vi "WebCam.Example03.vi"() -> ()   [LabVIEW 2021]
panel:
  out "snapshot 2":picture
  out "snapshot":picture
  in  "Case Constant\n(See Context Help)":bool
  in  "stop":bool
  out "error out":errorcluster
  in  "error in (no error)":errorcluster
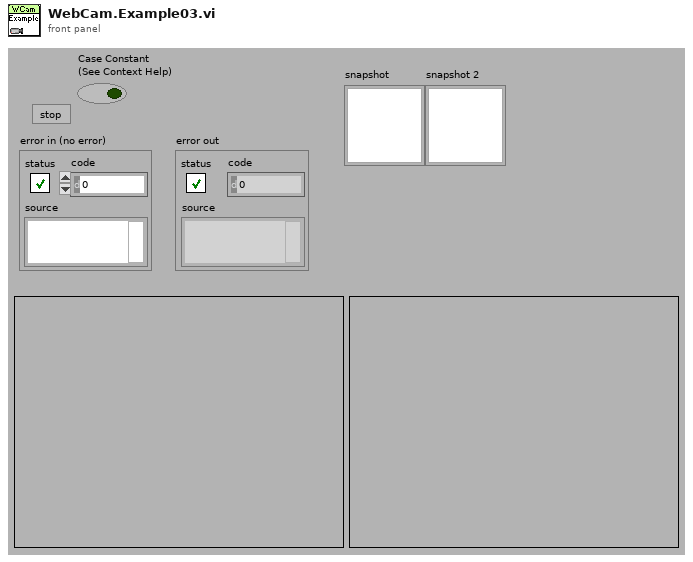
[diagram p1: front panel]
types:
  T1 = cluster{"posX":i32, "posY":i32, "nWidth":i32, "nHeight":i32}
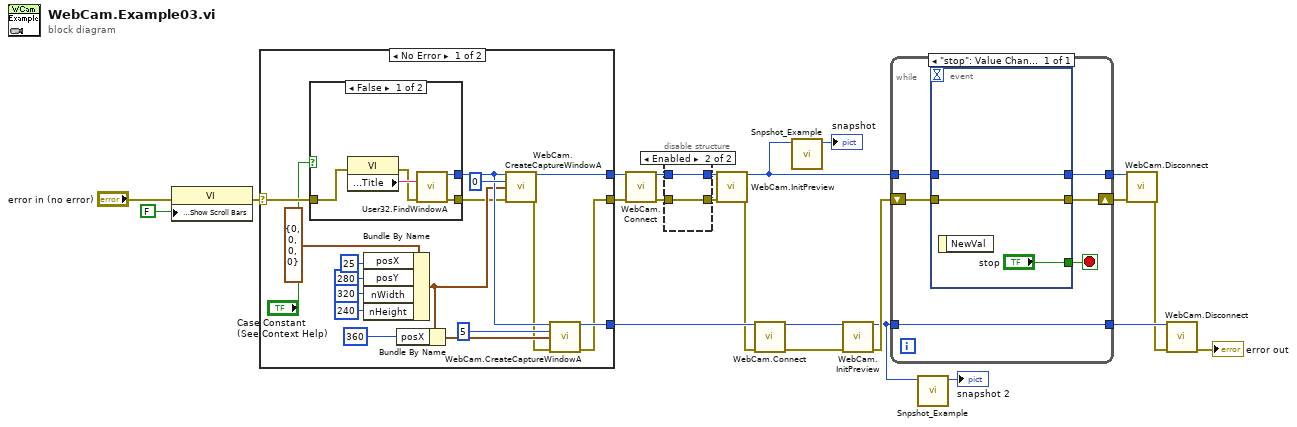
[diagram p0: block diagram]
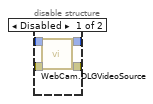
[diagram p2: hidden frame]
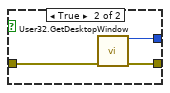
[diagram p3: hidden frame]
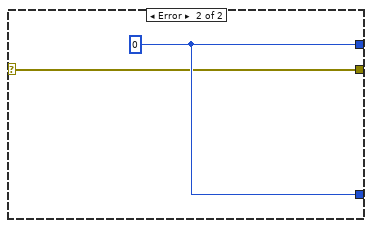
[diagram p4: hidden frame]
diagram:
  n1 = property class="VI"(error in="error in (no error)", "Front Panel Window:Show Scroll Bars"=FALSE) -> (error out=w20:errorcluster)  [unwired: 1 in, 1 out]
  n2 = case shown="No Error" w20 {
    selector: w20 -> [w40 w50]
    tunnel: [w41 w51] -> w15
    tunnel: [w24 w50] -> w14
    tunnel: [w30 w51] -> w18
    frame No Error {
      n3 = case shown="False" "Case Constant\n(See Context Help)" {
        tunnel: w40 -> [w43 w49]
        tunnel: [w46 w48] -> w33
        tunnel: [w45 w47] -> w25
        frame False {
          n4 = property class="VI"(error in=w43) -> (error out=w42:errorcluster, "Front Panel Window:Title"=w44:string)  [unwired: 1 in, 1 out]
          n5 = call "User32.FindWindowA.vi"("lpWindowName"=w44, "error in (no error)"=w42) -> ("hwnd"=w46:i32, "error out"=w45:errorcluster)  [unwired: 12 in]
        }
        frame True {
          n6 = call "User32.GetDesktopWindow.vi"("error in (no error)"=w49) -> ("Desktop handle"=w48:i32, "error out"=w47:errorcluster)  [unwired: 13 in]
        }
      }
      n7 = Bundle By Name(cluster=T1 {"posX"=0, "posY"=0, "nWidth"=0, "nHeight"=0} ("rect"), "posX"=25 ("nWidth"), "posY"=280 ("nWidth"), "nWidth"=320, "nHeight"=240 ("nWidth")) -> (w31:T1)
      n8 = Bundle By Name(cluster=w31, "posX"=360) -> (w28:T1)
      n9 = call "WebCam.CreateCaptureWindowA.vi"("handle"=w33, "nID"=0, "rect"=w31, "error in (no error)"=w25) -> ("handle out"=w41:i32, "error out"=w26:errorcluster)  [unwired: 10 in]
      n10 = call "WebCam.CreateCaptureWindowA.vi"("handle"=w33, "nID"=5, "rect"=w28, "error in (no error)"=w26) -> ("handle out"=w30:i32, "error out"=w24:errorcluster)  [unwired: 10 in]
    }
    frame Error {
      w51 = 0
    }
  }
  n11 = call "WebCam.Connect.vi"("handle"=w15, "error in (no error)"=w14) -> ("handle out"=w12:i32, "error out"=w11:errorcluster)  [unwired: 12 in]
  n12 = disable-structure shown="Enabled" {
    disable-tunnel: w12 -> [w55 w56]
    disable-tunnel: w11 -> [w54 w57]
    disable-tunnel: [w53 w57] -> w10
    disable-tunnel: [w52 w56] -> w9
    frame Disabled {
      n13 = call "WebCam.DLGVideoSource.vi"("handle"=w55, "error in (no error)"=w54) -> ("handle out"=w52:i32, "error out"=w53:errorcluster)  [unwired: 12 in]
    }
    frame Enabled {
    }
  }
  n14 = call "WebCam.InitPreview.vi"("handle"=w9, "error in (no error)"=w10) -> ("handle out"=w4:i32, "error out"=w8:errorcluster)  [unwired: 12 in]
  n15 = call "WebCam.Connect.vi"("handle"=w18, "error in (no error)"=w8) -> ("handle out"=w6:i32, "error out"=w5:errorcluster)  [unwired: 12 in]
  n16 = call "Snpshot_Example.vi"("handle"=w4) -> ("handle out"=→"snapshot":i32)  [unwired: 8 in, 2 out]
  n17 = call "WebCam.InitPreview.vi"("handle"=w6, "error in (no error)"=w5) -> ("handle out"=w1:i32, "error out"=w7:errorcluster)  [unwired: 12 in]
  n18 = while {
    shift-right: [w63] -> w23
    shift-left: w7 -> [w62]
    tunnel: w4 -> [w60]
    tunnel: [w59] -> w22
    tunnel: w1 -> [w58]
    tunnel: [w58] -> w17
    stop <- w61 stop-if-true
    n19 = event shown="[0] \"stop\": Value Change" {
      selector: _ -> [_]
      dyn-events: _ -> [_]
      timeout: _ -> [_]
      tunnel: [w66] -> w63
      tunnel: w62 -> [w66]
      tunnel: ["stop"] -> w61
      tunnel: w60 -> [w64]
      tunnel: [w64] -> w59
      event "stop": Value Change {
        n20 = event-data() -> ()  [unwired: 1 in, 1 out]
      }
    }
  }
  n21 = call "Snpshot_Example.vi"("handle"=w1) -> ("handle out"=→"snapshot 2":i32)  [unwired: 8 in, 2 out]
  n22 = call "WebCam.Disconnect.vi"("handle"=w22, "error in (no error)"=w23) -> ("error out"=w16:errorcluster)  [unwired: 13 in]
  n23 = call "WebCam.Disconnect.vi"("handle"=w17, "error in (no error)"=w16) -> ("error out"=→"error out":errorcluster)  [unwired: 13 in]
